vi "FilesList.vi"(11 "start path":path=path "") -> (0 "error out":errorcluster, 3 "Array":path[](array[path]))   [LabVIEW 2021, in "Tree.lvlib" / "Tree.lvclass"]
uses:
  Tree.lvclass
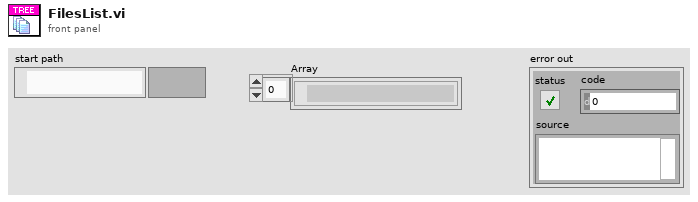
[diagram p1: front panel]
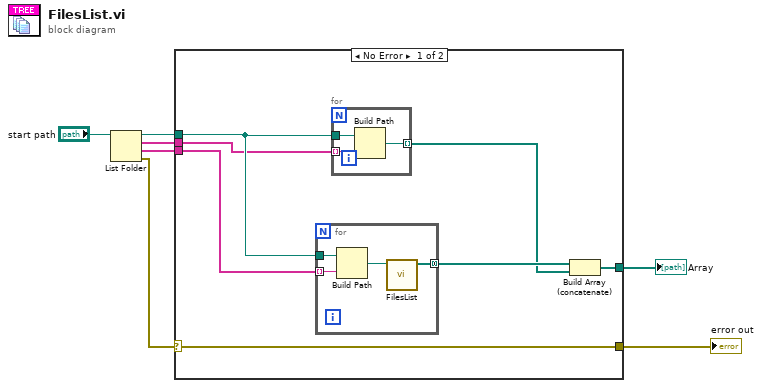
[diagram p0: block diagram]
diagram:
  n1 = List Folder(path="start path") -> (path out=w5:path, filenames=w4:string[], folder names=w6:string[], error out=w2:errorcluster)  [unwired: 3 in]
  n2 = case shown="No Error" w2 {
    selector: w2 -> [w8 w22]
    tunnel: w6 -> [w13 _]
    tunnel: w5 -> [w12 _]
    tunnel: w4 -> [w11 _]
    tunnel: [w10 _] -> w3
    tunnel: [w8 w22] -> w1
    frame No Error {
      n3 = for {
        tunnel: w12 -> [w21]
        tunnel: w13 -> [w20] mode=indexing
        tunnel: [w18] -> w14 mode=concatenating
        n4 = Build Path(base path=w21, name or relative path=w20) -> (appended path=w19:path)
        n5 = call "FilesList.vi"("start path"=w19) -> ("Array"=w18:path[])  [unwired: 9 in, 1 out]
      }
      n6 = for {
        tunnel: w12 -> [w17]
        tunnel: w11 -> [w16] mode=indexing
        tunnel: [w15] -> w9 mode=indexing
        n7 = Build Path(base path=w17, name or relative path=w16) -> (appended path=w15:path)
      }
      n8 = Build Array (concatenate)(w14, w9) -> (w10:path[])
    }
    frame Error {
    }
  }
  "Array" <- w3
  "error out" <- w1
